vi "Leap Circle Gesture Progress.vi"() -> ()   [LabVIEW 2011, in "LVH-Leap.lvlib"]
doc: "This example demonstrates how to read the progress of a circle gesture using the Leap Motion Controller."
uses:
  vi.lib/LabVIEW Hacker/Leap/LVH-Leap.lvlib
  vi.lib/LabVIEW Hacker/Leap/Public/Gestures/Circle/Instance VIs/Read 1 Circle Progress.vi
panel:
  out "Circle Gesture Progress":dbl(knob) scale=0.0..20.0
  in  "Stop Button":bool
  # "Circle Gesture Progress Example\n\nThis example demonstrates how to read the progress of a circle gesture \nusing the Leap Motion Controller.\n\nInstructions\n1. Connect the Leap Motion Controller to the host computer.\n2. Click the Run Arrow.\n3. Make a circle motion above the Leap and notice the gauge value increase."
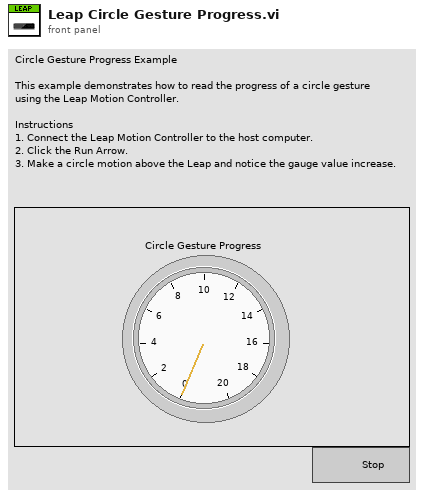
[diagram p1: front panel]
types:
  T1 = typedef "LVH-Leap.lvlib/Leap Handle.ctl" = cluster{"LeapCSharp":refnum<k24>}
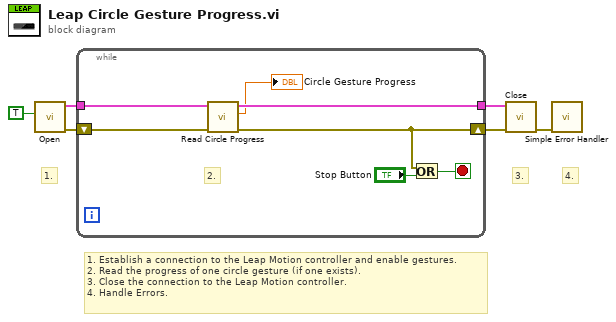
[diagram p0: block diagram]
diagram:
  # "1. Establish a connection to the Leap Motion controller and enable gestures.\n2. Read the progress of one circle gesture (if one exists).\n3. Close the connection to the Leap Motion controller.\n4. Handle Errors."
  # "4."
  # "3."
  # "1."
  n1 = call "Open.vi"("Enable Gestures? (T)"=TRUE) -> ("Error Out"=w4:errorcluster, "Leap Handle"=w6:T1)  [unwired: 9 in]
  n2 = while {
    tunnel: w6 -> [w10]
    shift-right: [w7] -> w5
    shift-left: w4 -> [w11]
    tunnel: [w9] -> w2
    stop <- w13 stop-if-true
    # "2."
    n3 = call-poly "Read Circle Progress.vi"("Error In"=w11, "Leap Handle"=w10) -> ("Error Out"=w7:errorcluster, "Circle Progress"=→"Circle Gesture Progress":dbl, "Leap Handle"=w9:T1)  [unwired: 6 in, 1 out]
    n4 = Or(x=w7, y="Stop Button") -> (x .or. y?=w13:bool)
  }
  n5 = call "Close.vi"("Error In"=w5, "Leap Handle"=w2) -> ("Error Out"=w1:errorcluster)  [unwired: 9 in]
  n6 = call <vilib>:"Simple Error Handler.vi"("error in (no error)"=w1) -> ()  [unwired: 4 in, 5 out]
